vi "LED off.vi"() -> ()   [LabVIEW 2019]
panel:
  out "LED Strip":u32[](array[colorbox])
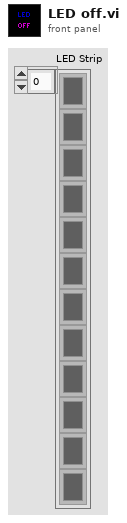
[diagram p1: front panel]
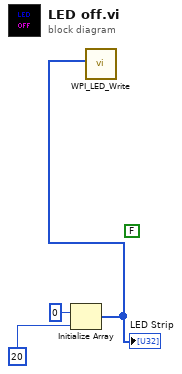
[diagram p0: block diagram]
diagram:
  (unwired) FALSE
  n1 = Initialize Array(u32 0 ("element"), 20 ("dimension size")) -> (w1:u32[])
  "LED Strip" <- w1
  n2 = call <vilib>:"WPI_LED_Write.vi"("Color Array"=w1) -> ()  [unwired: 10 in, 1 out]
